vi "GenINI_Read_Original_INI.vi"(8 "error in (no error)":errorcluster, 10 "Guess types?":bool, 11 "Path":path=path "C:/Documents and Settings/joseph.zoller/Desktop/LV_INI/test.ini") -> (0 "error out":errorcluster, 3 "Value types":T1[](array[typedef]))   [LabVIEW 2009]
uses:
  Typedefs/GenINI_Key_Values.ctl
  Typedefs/GenINI_Read_Types.ctl
  <vilib>/Utility/config.llb/Read Key (String).vi
  <vilib>/Utility/config.llb/NI_LVConfig.lvlib
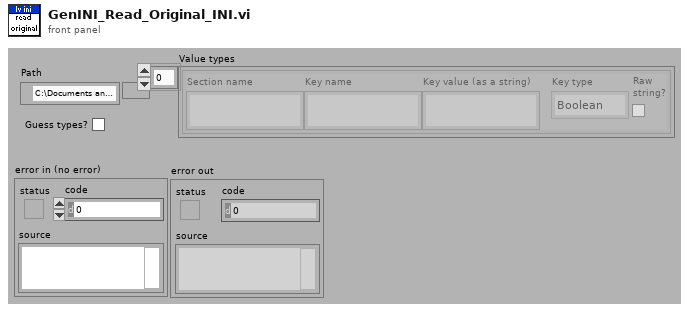
[diagram p1: front panel]
types:
  T1 = typedef "GenINI_Key_Values.ctl" = cluster{"Section name":string, "Key name":string, "Key value (as a string)":string, "Key type":T2, "Raw\nstring?":bool}
  T2 = typedef "GenINI_Read_Types.ctl" = enum16{"Boolean", "Double", "I32", "Path", "String", "U32"}
  T3 = typedef "NI_LVConfig.lvlib/Config Data RefNum.ctl" = refnum<k1>
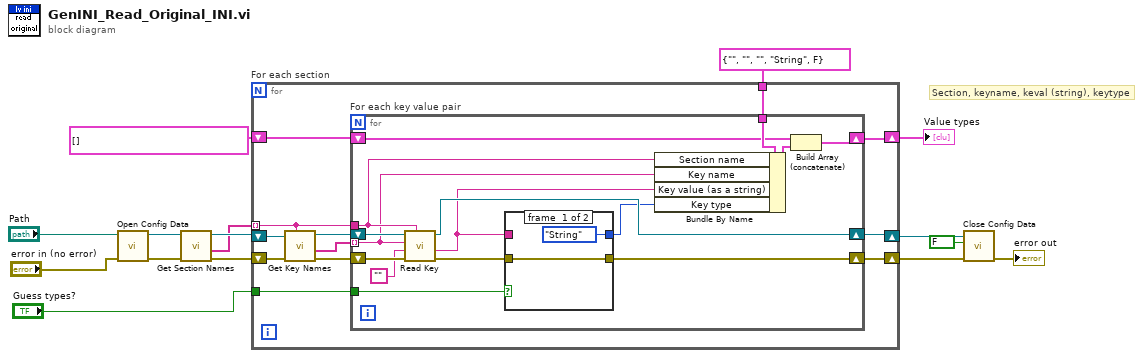
[diagram p0: block diagram]
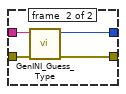
[diagram p2: hidden frame]
diagram:
  # "Section, keyname, keval (string), keytype"
  n1 = call <vilib>:"Open Config Data.vi"("error in (no error)"="error in (no error)", "configuration file path"="Path") -> ("error out"=w13:errorcluster, "refnum"=w12:T3)  [unwired: 7 in, 1 out]
  n2 = call <vilib>:"Get Section Names.vi"("error in (no error)"=w13, "refnum"=w12) -> ("error out"=w10:errorcluster, "section names"=w9:string[], "refnum out"=w11:T3)  [unwired: 7 in]
  n3 = for "For each section" {
    shift-right: [w23] -> w6
    shift-left: w11 -> [w26]
    shift-right: [w22] -> w8
    shift-left: w10 -> [w27]
    tunnel: w9 -> [w20] mode=indexing
    shift-right: [w19] -> w2
    shift-left: T1[] [] -> [w17]
    tunnel: T1 {"Section name"="", "Key name"="", "Key value (as a string)"="", "Key type"=enum."String", "Raw\nstring?"=FALSE} ("INI values") -> [w18]
    tunnel: "Guess types?" -> [w16]
    n4 = call <vilib>:"Get Key Names.vi"("section"=w20, "error in (no error)"=w27, "refnum"=w26) -> ("error out"=w25:errorcluster, "key names"=w21:string[], "refnum out"=w24:T3)  [unwired: 5 in, 1 out]
    n5 = for "For each key value pair" {
      shift-right: [w40] -> w23
      shift-left: w24 -> [w41]
      shift-right: [w29] -> w22
      shift-left: w25 -> [w42]
      tunnel: w21 -> [w34] mode=indexing
      tunnel: w20 -> [w35]
      shift-right: [w36] -> w19
      shift-left: w17 -> [w37]
      tunnel: w18 -> [w39]
      tunnel: w16 -> [w28]
      n6 = call-poly <vilib>:"Read Key.vi"("section"=w35, "error in (no error)"=w42, "default value"="", "key"=w34, "refnum"=w41) -> ("error out"=w30:errorcluster, "value"=w32:string, "refnum out"=w40:T3)  [unwired: 3 in, 1 out]
      n7 = case shown="False" w28 {
        tunnel: w32 -> [_ w48]
        tunnel: [GenINI_Read_Types."String" ("Guessed type") w47] -> w31
        tunnel: w30 -> [w43 w46]
        tunnel: [w43 w45] -> w29
        frame #0 {
        }
        frame #1 {
          n8 = call "GenINI_Guess_Type.vi"("error in (no error)"=w46, "key value"=w48) -> ("error out"=w45:errorcluster, "Guessed type"=w47:T2)  [unwired: 8 in]
        }
      }
      n9 = Bundle By Name(cluster=w39, "Section name"=w35, "Key name"=w34, "Key value (as a string)"=w32, "Key type"=w31) -> (w38:T1)
      n10 = Build Array (concatenate)(w37, w38) -> (w36:T1[])
    }
  }
  "Value types" <- w2
  n11 = call <vilib>:"Close Config Data.vi"("error in (no error)"=w8, "write file if changed (T)"=FALSE, "refnum"=w6) -> ("error out"=→"error out":errorcluster)  [unwired: 7 in, 1 out]
